vi "configuration UI.vi"() -> ()   [LabVIEW 2013, in "Scaling editor node.lvclass"]
uses:
  Scaling editor node.lvclass
  <vilib>/NI/Configuration Framework/Node/NodeRef.ctl
  <vilib>/NI/Configuration Framework/Node/NISE_CEF_Node.lvclass
  <vilib>/NI/AMC/Message Queue.ctl
  <vilib>/NI/AMC/Message.ctl
  <vilib>/NI/Tools/Keyed Array/KeyedArray.ctl
  <vilib>/NI/Configuration Framework/Node/UserEventRef.ctl
  <vilib>/NI/Configuration Framework/Controls/EventCluster.ctl
  <vilib>/NI/Configuration Framework/Node/StopEvent.ctl
  <vilib>/NI/Configuration Framework/Node/RefreshUIEvent.ctl
  <vilib>/NI/Configuration Framework/Node/CacheState.ctl
  <vilib>/NI/Configuration Framework/Node/NodeChangeEvent.ctl
  System.Windows.Forms
  module/configuration/controls/scale data types.ctl
  <vilib>/NI/DCAF Table API/Table Manager/references.ctl
  <vilib>/NI/Tag Bus Data Framework/control module/editor node/channel action event.ctl
  <vilib>/NI/Tag Bus Data Framework/control module/editor node/dialog output action.ctl
  <vilib>/NI/Tag Bus Module Framework/channel/TBM channel.lvclass
  <vilib>/NI/Tag Bus/tag/tag descriptor.lvclass
  <vilib>/NI/DCAF Table API/Listbox/Multi Column Listbox.lvclass
  <vilib>/NI/DCAF Table API/Listbox/Multi Column Listbox.lvclass/Multi Column Listbox.ctl
  <vilib>/NI/DCAF Table API/Table Manager/Table Manager.lvclass/Table Manager.ctl
  <vilib>/NI/DCAF Table API/Data Grid/Data Grid.lvclass
  <vilib>/NI/DCAF Table API/Listbox/Write Listbox.vi
  <vilib>/NI/DCAF Table API/Table Manager/Write Top VI.vi
  <vilib>/NI/Tag Bus Data Framework/control module/editor node/control module editor.lvclass
  <vilib>/NI/Tools/Keyed Array/Tools_KeyedArray.lvlib
  <vilib>/NI/AMC/AMC.lvlib
  <vilib>/NI/Configuration Framework/NISE_CEF_TreeControl.lvlib
  <vilib>/NI/DCAF Table API/Table Manager/Table Manager.lvclass
  module/configuration/Scaling configuration.lvclass
panel:
  in  "Remove Scale":bool
  in  "Add Scale":bool
  in  "scale data types":T1
  in  "Scales":i32(listbox)
  in  "node change":T2
  in  "cache state":T3
  in  "refresh UI":T4
  in  "stop event":T5
  in  "Tab Control":T6(tab)
  in  "DataGridView":refnum<k24>(container)
  in  "Remove Mapping":bool
  in  "Add Mapping":bool
  in  "Multicolumn Listbox":i32(listbox)
  in  "user event":T7
  in  "main queue":T8
  in  "node ref":T9
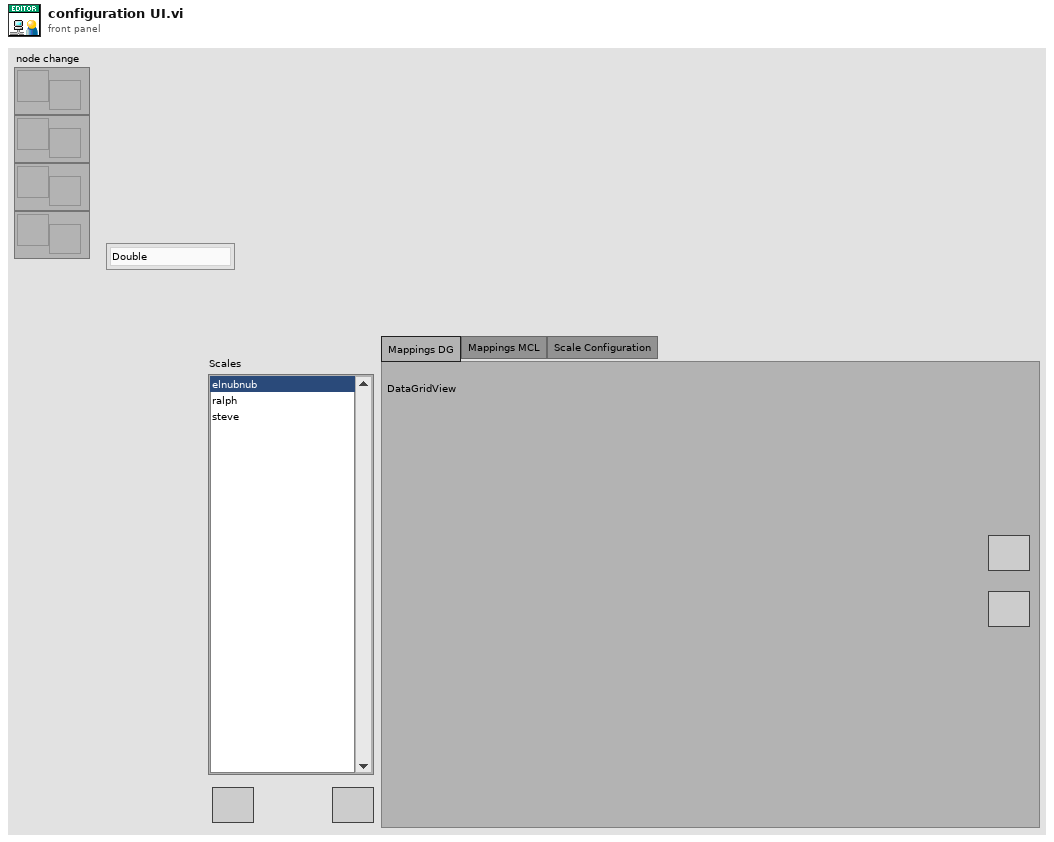
[diagram p1: front panel]
types:
  T1 = typedef "Scaling configuration.lvclass/scale data types.ctl" = enum16{"Double", "Single", "I64", "I32", "I16", "I8", "U64", "U32", "U16", "U8"}
  T2 = typedef "NISE_CEF_Node.lvclass/NodeChangeEvent.ctl" = refnum<user-event>
  T3 = typedef "NISE_CEF_Node.lvclass/CacheState.ctl" = refnum<user-event>
  T4 = typedef "NISE_CEF_Node.lvclass/RefreshUIEvent.ctl" = refnum<user-event>
  T5 = typedef "NISE_CEF_Node.lvclass/StopEvent.ctl" = refnum<user-event>
  T6 = enum32{"Mappings DG", "Mappings MCL", "Scale Configuration"}
  T7 = typedef "NISE_CEF_Node.lvclass/UserEventRef.ctl" = refnum<user-event>
  T8 = typedef "AMC.lvlib/Message Queue.ctl" = refnum<queue>
  T9 = typedef "NISE_CEF_Node.lvclass/NodeRef.ctl" = refnum<data-value>
  T10 = typedef "Table Manager.lvlib/Table Manager.lvclass/references.ctl" = cluster{"stop event":T5, "refresh UI":T4, "cache state":T3, "node change":T2, "user event out":refnum<user-event>, "main queue":T8, "user event":T7}
  T11 = typedef "Table Manager.lvlib/Table Manager.lvclass/object ref.ctl" = cluster{"engine":refnum<data-value>, "Node Ref":refnum<data-value>}
  T12 = typedef "Table Manager.lvlib/Column.lvclass/Column Descriptor.ctl" = cluster{"name":string, "caption":string, "Column Type":T13, "Params":string, "AutoSizeMode":i32, "FillWeight":sgl, "MinWidth":u32, "tooltip":string, "Enum Reference":refnum<vi>, "Channel suffix":string, "Read Only":bool, "Call Back VI":T14, "DT Dependency":i32, "name dependency":i32, "data type":T15}
  T13 = typedef "Table Manager.lvlib/Column.lvclass/Column Type.ctl" = enum16{"String", "Mapping", "Channel Name", "Tag", "Enum", "Data Type", "Numeric"}
  T14 = typedef "Table Manager.lvlib/Table Manager.lvclass/Call Back Ref Type Def.ctl" = refnum<vi>
  T15 = typedef "tag bus.lvlib/tag descriptor.lvclass/Data Type.ctl" = enum16{"Double", "Single", "I64", "I32", "I16", "I8", "U64", "U32", "U16", "U8", "Boolean", "String", "Array of Double", "Array of Single", "Array of I64", "Array of I32", "Array of I16", "Array of I8", "Array of U64", "Array of U32", "Array of U16", "Array of U8", "Array of Boolean", "Array of String"}
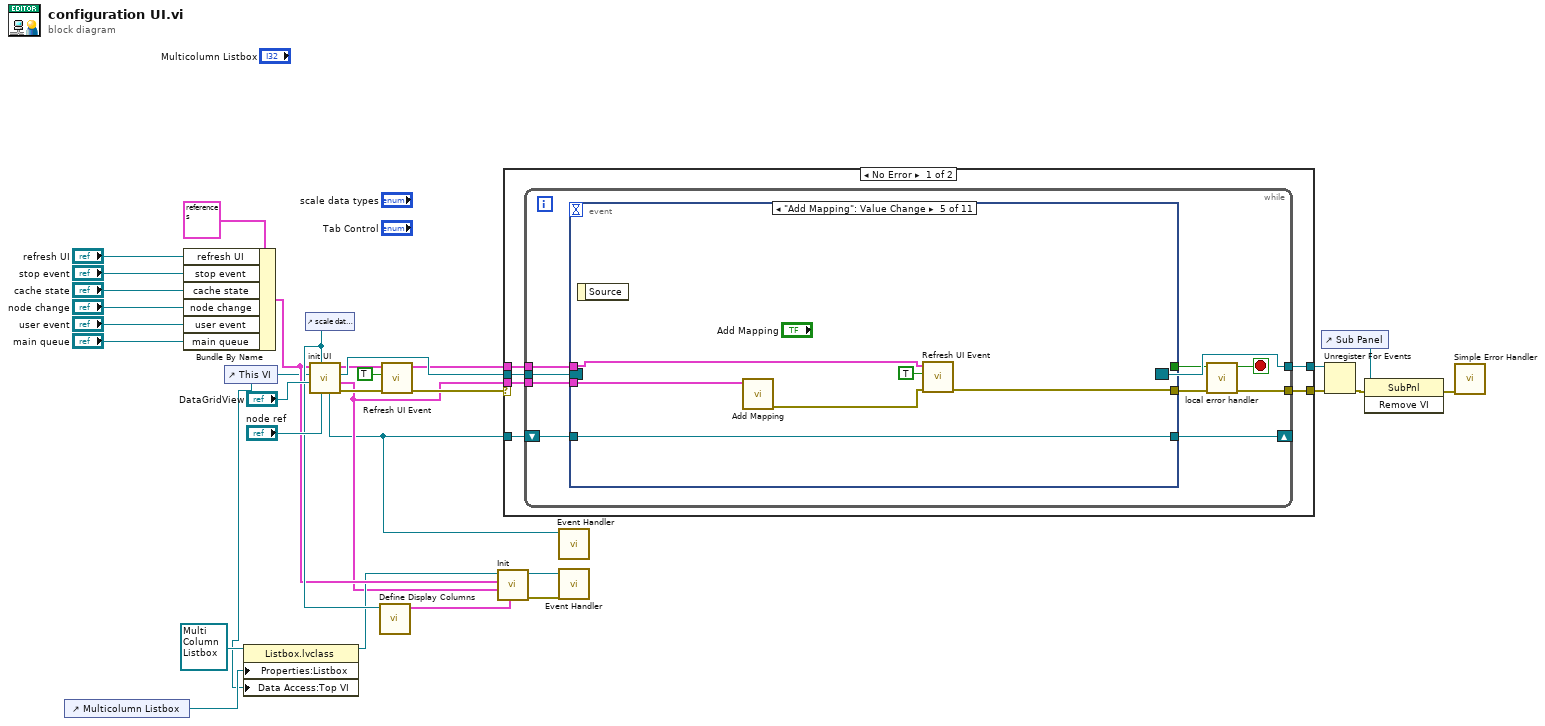
[diagram p0: block diagram]
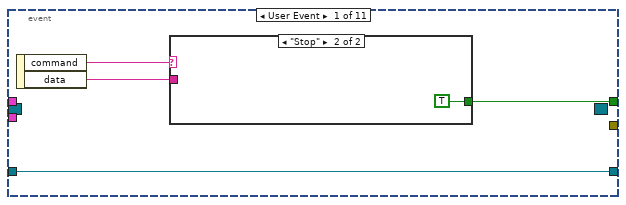
[diagram p2: hidden frame]
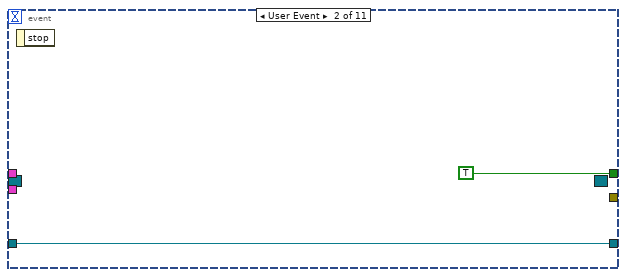
[diagram p4: hidden frame]
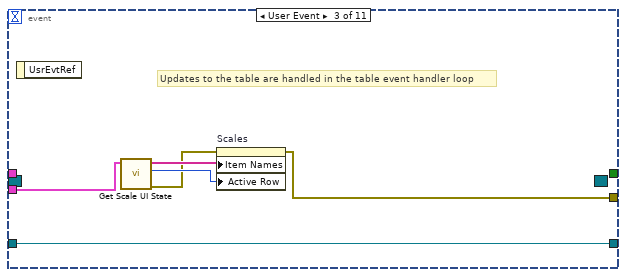
[diagram p5: hidden frame]
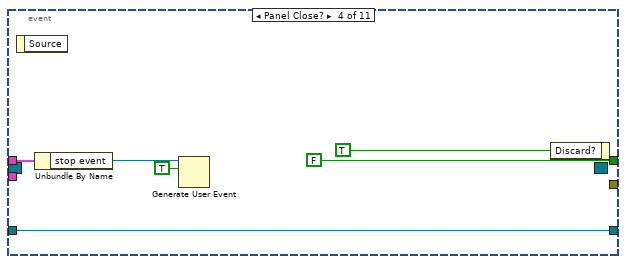
[diagram p6: hidden frame]
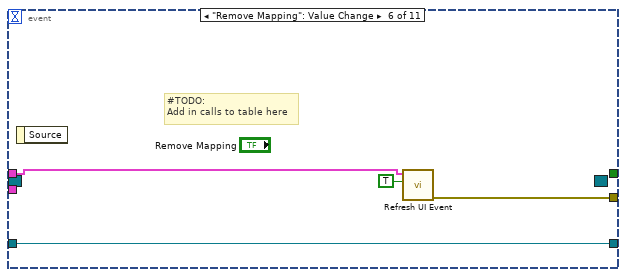
[diagram p7: hidden frame]
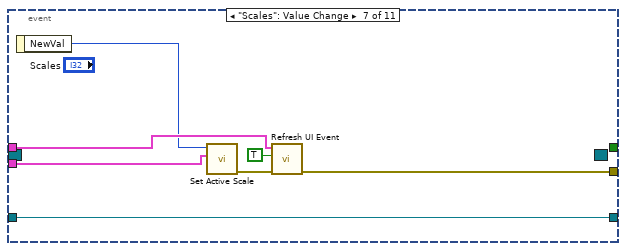
[diagram p8: hidden frame]
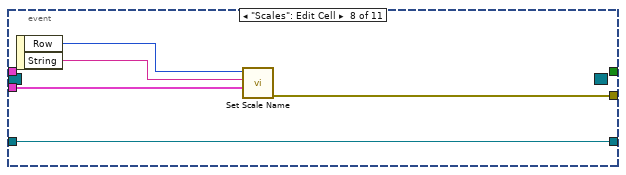
[diagram p9: hidden frame]
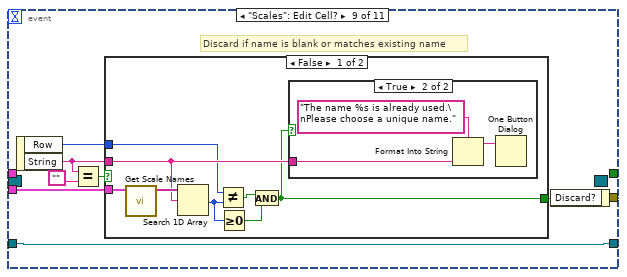
[diagram p10: hidden frame]
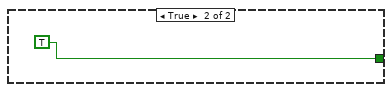
[diagram p12: hidden frame]
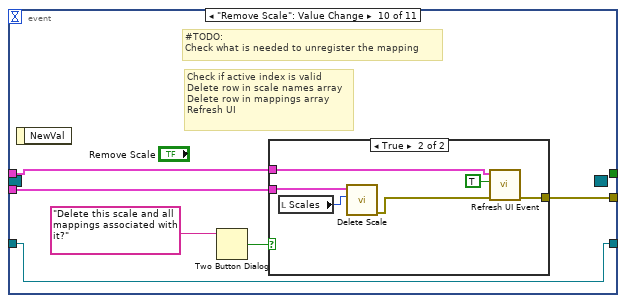
[diagram p13: hidden frame]
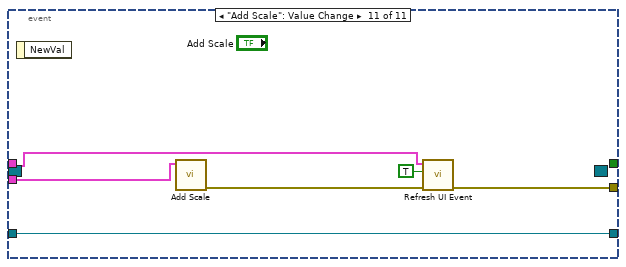
[diagram p15: hidden frame]
diagram:
  n1 = control-ref of="Multicolumn Listbox"() -> (w10:refnum<vi>)
  n2 = Bundle By Name(cluster=T10 {"stop event"=refnum, "refresh UI"=refnum, "cache state"=refnum, "node change"=refnum, "user event out"=refnum, "main queue"=refnum, "user event"=refnum} ("References in"), "refresh UI"="refresh UI", "stop event"="stop event", "cache state"="cache state", "node change"="node change", "user event"="user event", "main queue"="main queue") -> (w12:T10)
  n3 = control-ref of="This VI"() -> (w9:refnum<vi>)
  n4 = property class="Listbox.lvclass"(reference=refnum<class "Multi Column Listbox.lvclass"> refnum ("Multi Column Listbox in"), "Properties:Listbox"=w10, "Data Access:Top VI"=w9) -> (reference out=w8:refnum<class "Multi Column Listbox.lvclass">)  [unwired: 1 in, 1 out]
  n5 = control-ref of="scale data types"() -> (w13:refnum<vi>)
  n6 = call "init UI.vi"("node ref"="node ref", "scale data types"=w13, ".NET Refnum in"="DataGridView", "This VI"=w9, "References in"=w12) -> ("error out"=w15:errorcluster, "Objects out"=w7:T11, "Event Registration Refnum"=w21:refnum<event-registration>, "References out"=w18:T10, "Data Grid out"=w6:refnum<class "Data Grid.lvclass">)  [unwired: 2 in]
  n7 = call "Define Display Columns.vi"("Enum in"=w13) -> ("Columns"=w14:T12[])  [unwired: 10 in]
  n8 = call "Refresh UI Event.vi"("error in"=w15, "Refresh?"=TRUE, "References in"=w18) -> ("error out"=w20:errorcluster, "References out"=w17:T10)  [unwired: 7 in]
  n9 = call-dynamic "Init.vi"("Column Definitions"=w14, "object refs"=w7, "References in"=w12, "Multi Column Listbox in"=w8) -> ("error out"=w4:errorcluster, "Multi Column Listbox out"=w5:refnum<class "Multi Column Listbox.lvclass">)  [unwired: 5 in, 1 out]
  n10 = case shown="No Error" w20 {
    selector: w20 -> [_ w127]
    tunnel: w21 -> [w37 w126]
    tunnel: [w36 w126] -> w31
    tunnel: [w35 w127] -> w30
    tunnel: w7 -> [w33 _]
    tunnel: w17 -> [w34 _]
    tunnel: w6 -> [w32 _]
    frame No Error {
      n11 = while {
        tunnel: w37 -> [w47]
        tunnel: [w46] -> w36
        tunnel: [w43] -> w35
        tunnel: w34 -> [w42]
        tunnel: w33 -> [w41]
        shift-right: [w39] -> _
        shift-left: w32 -> [w40]
        stop <- w45 stop-if-true
        n12 = event shown="[4] \"Add Mapping\": Value Change" {
          selector: w47 -> [_ _ _ _ _ _ _ _ _ _ _]
          dyn-events: [_ _ _ _ _ _ _ _ _ _ _] -> w46
          timeout: _ -> [_ _ _ _ _ _ _ _ _ _ _]
          tunnel: [w51 TRUE _ FALSE _ _ _ _ _ _ _] -> w44
          tunnel: w42 -> [_ _ _ w63 w70 w74 w81 _ _ w112 w124]
          tunnel: w41 -> [_ _ w55 _ w68 _ w78 w86 w93 w109 w122]
          tunnel: w40 -> [w48 w53 w60 w61 w69 w73 w77 w84 w90 w108 w120]
          tunnel: [w48 w53 w60 w61 w69 w73 w77 w84 w90 w108 w120] -> w39
          tunnel: [_ _ w56 _ w72 w76 w83 w85 _ w113 w123] -> w38
          event User Event {
            n13 = event-data() -> ("command"=w50:string, "data"=w49:string)  [unwired: 1 in]
            n14 = case shown="\"Stop\"" w50 {
              tunnel: [_ TRUE] -> w51
              tunnel: w49 -> [_ _]
              frame Default {
              }
              frame "Stop" {
              }
            }
          }
          event User Event {
            n15 = event-data() -> ()  [unwired: 1 in, 1 out]
          }
          event User Event {
            # "Updates to the table are handled in the table event handler loop"
            n16 = event-data() -> ()  [unwired: 1 in, 1 out]
            n17 = call "Get Scale UI State.vi"("references"=w55) -> ("error out"=w57:errorcluster, "active scale index"=w58:i32, "scale names"=w59:string[])  [unwired: 8 in]
            n18 = property on="Scales" class="LstBox (strict)"(error in=w57, "Item Names"=w59, "Active Row"=w58) -> (error out=w56:errorcluster)  [unwired: 1 in, 1 out]
          }
          event Panel Close? {
            n19 = event-data() -> ()  [unwired: 1 in, 1 out]
            n20 = Unbundle By Name(w63) -> ("stop event"=w62:T5)
            n21 = Generate User Event(user event=w62, event data cluster=TRUE ("event data")) -> ()  [unwired: 2 in, 2 out]
            n22 = event-data("Discard?"=TRUE) -> ()  [unwired: 1 in, 1 out]
          }
          event "Add Mapping": Value Change {
            n23 = event-data() -> ()  [unwired: 1 in, 1 out]
            n24 = call "Add Mapping.vi"("references"=w68) -> ("error out"=w67:errorcluster)  [unwired: 9 in, 1 out]
            n25 = call "Refresh UI Event.vi"("error in"=w67, "Refresh?"=TRUE, "References in"=w70) -> ("error out"=w72:errorcluster)  [unwired: 7 in, 1 out]
          }
          event "Remove Mapping": Value Change {
            # "#TODO:\nAdd in calls to table here"
            n26 = event-data() -> ()  [unwired: 1 in, 1 out]
            n27 = call "Refresh UI Event.vi"("Refresh?"=TRUE, "References in"=w74) -> ("error out"=w76:errorcluster)  [unwired: 8 in, 1 out]
          }
          event "Scales": Value Change {
            n28 = event-data() -> ("NewVal"=w80:i32)  [unwired: 1 in]
            n29 = call "Set Active Scale.vi"("references"=w78, "Index"=w80) -> ("error out"=w82:errorcluster)  [unwired: 9 in]
            n30 = call "Refresh UI Event.vi"("error in"=w82, "Refresh?"=TRUE, "References in"=w81) -> ("error out"=w83:errorcluster)  [unwired: 7 in, 1 out]
          }
          event "Scales": Edit Cell {
            n31 = event-data() -> ("Row"=w88:i32, "String"=w87:string)  [unwired: 1 in]
            n32 = call "Set Scale Name.vi"("references"=w86, "name"=w87, "index"=w88) -> ("error out"=w85:errorcluster)  [unwired: 8 in]
          }
          event "Scales": Edit Cell? {
            # "Discard if name is blank or matches existing name"
            n33 = event-data() -> ("Row"=w89:i32, "String"=w92:string)  [unwired: 1 in]
            n34 = Equal?(x=w92, y="") -> (x = y?=w95:bool)
            n35 = case shown="False" w95 {
              tunnel: [w96 TRUE] -> w94
              tunnel: w93 -> [w103 _]
              tunnel: w92 -> [w101 _]
              tunnel: w89 -> [w100 _]
              frame False {
                n36 = call "Get Scale Names.vi"("references"=w103) -> ("scale names"=w102:string[])  [unwired: 9 in, 1 out]
                n37 = Search 1D Array(1D array=w102, element=w101) -> (index of element=w99:i32)  [unwired: 1 in]
                n38 = Not Equal?(x=w100, y=w99) -> (x != y?=w98:bool)
                n39 = Greater Or Equal To 0?(x=w99) -> (x >= 0?=w97:bool)
                n40 = And(x=w98, y=w97) -> (x .and. y?=w96:bool)
                n41 = case shown="True" w96 {
                  tunnel: w101 -> [_ w104]
                  frame False {
                  }
                  frame True {
                    n42 = Format Into String(format string="The name %s is already used.\nPlease choose a unique name.", w104) -> (resulting string=w106:string)  [unwired: 2 in, 1 out]
                    n43 = One Button Dialog(message=w106) -> ()  [unwired: 1 in, 1 out]
                  }
                }
              }
              frame True {
              }
            }
            n44 = event-data("Discard?"=w94) -> ()  [unwired: 1 in, 1 out]
          }
          event "Remove Scale": Value Change {
            # "#TODO:\nCheck what is needed to unregister the mapping"
            # "Check if active index is valid\nDelete row in scale names array\nDelete row in mappings array\nRefresh UI"
            n45 = event-data() -> ()  [unwired: 1 in, 1 out]
            n46 = Two Button Dialog(message="Delete this scale and all mappings associated with it?" ("format string")) -> (T button?=w110:bool)  [unwired: 2 in]
            n47 = case shown="True" w110 {
              tunnel: [_ w119] -> w113
              tunnel: w112 -> [_ w117]
              tunnel: w109 -> [_ w116]
              frame False {
              }
              frame True {
                n48 = local read "Scales"() -> (w115:i32)
                n49 = call "Delete Scale.vi"("Index"=w115, "references"=w116) -> ("error out"=w114:errorcluster)  [unwired: 9 in]
                n50 = call "Refresh UI Event.vi"("error in"=w114, "Refresh?"=TRUE, "References in"=w117) -> ("error out"=w119:errorcluster)  [unwired: 7 in, 1 out]
              }
            }
          }
          event "Add Scale": Value Change {
            n51 = event-data() -> ()  [unwired: 1 in, 1 out]
            n52 = call "Add Scale.vi"("references"=w122) -> ("error out"=w121:errorcluster)  [unwired: 10 in]
            n53 = call "Refresh UI Event.vi"("error in"=w121, "Refresh?"=TRUE, "References in"=w124) -> ("error out"=w123:errorcluster)  [unwired: 7 in, 1 out]
          }
        }
        n54 = call "local error handler.vi"("error in (no error)"=w38, "Boolean in"=w44) -> ("error out"=w43:errorcluster, "Boolean out"=w45:bool)  [unwired: 8 in]
      }
    }
    frame Error {
    }
  }
  n55 = call-dynamic "Event Handler.vi"("Data Grid in"=w6) -> ()  [unwired: 9 in, 2 out]
  n56 = call-dynamic "Event Handler.vi"("error in"=w4, "Listbox in"=w5) -> ()  [unwired: 8 in, 2 out]
  n57 = control-ref of="Sub Panel"() -> (w3:refnum<vi>)
  n58 = Unregister For Events(event registration refnum=w31, error in=w30) -> (error out=w2:errorcluster)
  n59 = invoke class="SubPnl" method="Remove VI"(reference=w3, error in=w2) -> (error out=w1:errorcluster)  [unwired: 1 in, 2 out]
  n60 = call <vilib>:"Simple Error Handler.vi"("error in (no error)"=w1) -> ()  [unwired: 4 in, 5 out]
